vi "PXI-Execute Pause.vi"(9 "Pause?":bool, 11 "error in (no error)":errorcluster) -> (8 "Abort":bool, 15 "error out":errorcluster)   [LabVIEW 2015]
uses:
  PXI Globals.vi
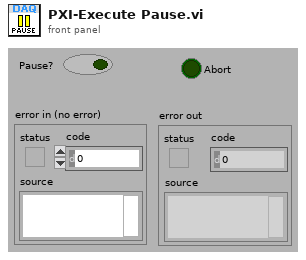
[diagram p1: front panel]
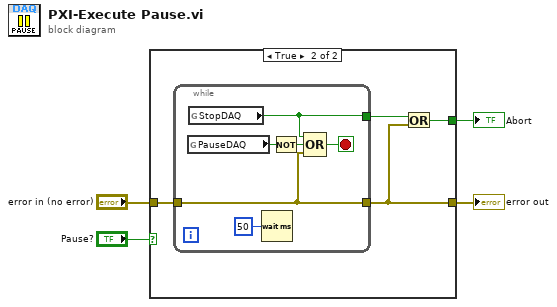
[diagram p0: block diagram]
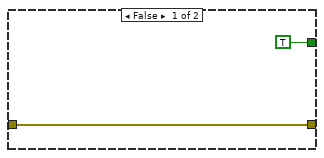
[diagram p2: hidden frame]
diagram:
  n1 = case shown="True" "Pause?" {
    tunnel: [w6 w7] -> w4
    tunnel: "error in (no error)" -> [w6 w8]
    tunnel: [TRUE w9] -> w2
    frame False {
    }
    frame True {
      n2 = while {
        tunnel: w8 -> [w11]
        tunnel: [w11] -> w7
        tunnel: [w12] -> w10
        stop <- w16 stop-if-true
        n3 = global read "PXI Globals.vi" "PauseDAQ"() -> (w15:bool)
        n4 = global read "PXI Globals.vi" "StopDAQ"() -> (w12:bool)
        n5 = Wait (ms)(milliseconds to wait=u32 50) -> ()  [unwired: 1 out]
        n6 = Not(x=w15) -> (.not. x?=w14:bool)
        n7 = Compound Arithmetic op=OR(w12, w14, w11) -> (w16:bool)
      }
      n8 = Or(x=w10, y=w7) -> (x .or. y?=w9:bool)
    }
  }
  "error out" <- w4
  "Abort" <- w2
